vi "LB_SetCaptureGain.vi"(9 "Gain":u8=1 min=1 max=4, 10 "SamplingTime":T1, 11 "LB_COM_IN":refnum<visa-resource-name>="COM4") -> (2 "OK":bool)   [LabVIEW 2015, in "LBAnalyser.lvlib"]
uses:
  LBAnalyser.lvlib
  SamplingTime.ctl
  UartCOM/UARTCOM.lvlib
panel:
  out "error out":errorcluster caption="错误输出"
  in  "error in (no error)":errorcluster caption="错误输入（无错误）"
  # "1~4"
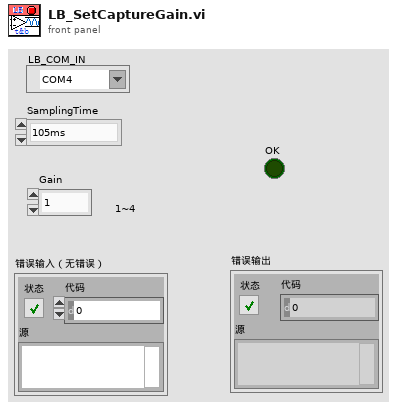
[diagram p1: front panel]
types:
  T1 = typedef "LBAnalyser.lvlib/SamplingTime.ctl" = enum8{"105ms", "120ms", "165ms", "270ms", "380ms", "880ms"}
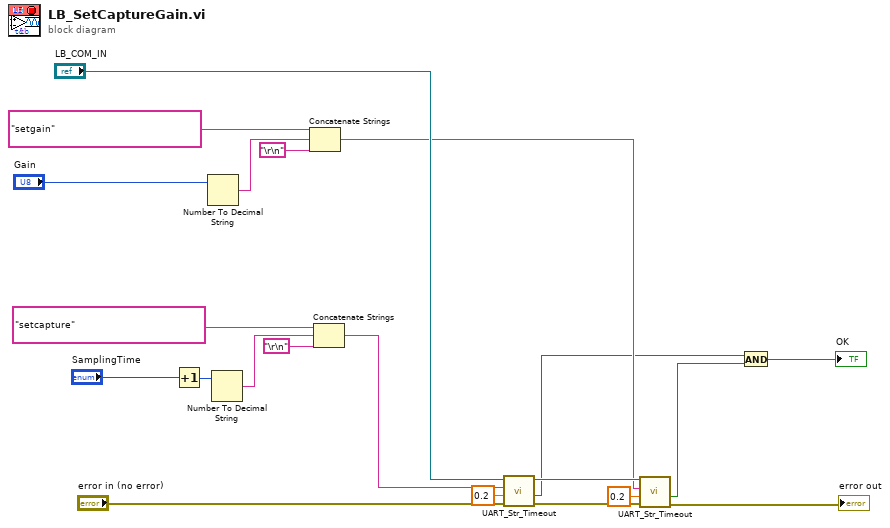
[diagram p0: block diagram]
diagram:
  n1 = Increment(x="SamplingTime") -> (x+1=w18:T1)
  n2 = Number To Decimal String(number="Gain") -> (decimal integer string=w12:string)  [unwired: 1 in]
  n3 = Number To Decimal String(number=w18) -> (decimal integer string=w16:string)  [unwired: 1 in]
  n4 = Concatenate Strings("setgain" ("写入字符串"), w12, "\r\n") -> (w5:string)
  n5 = Concatenate Strings("setcapture" ("写入字符串"), w16, "\r\n") -> (w14:string)
  n6 = call "UART_Str_Timeout.vi"("error in (no error)"="error in (no error)", "超时s"=0.2, "写入字符串"=w14, "BASE_COM"="LB_COM_IN") -> ("error out"=w7:errorcluster, "OK"=w3:bool, "BASE_COM_OUT"=w6:refnum<visa-resource-name>)  [unwired: 3 in, 2 out]
  n7 = call "UART_Str_Timeout.vi"("error in (no error)"=w7, "超时s"=0.2, "写入字符串"=w5, "BASE_COM"=w6) -> ("error out"=→"error out":errorcluster, "OK"=w2:bool)  [unwired: 3 in, 3 out]
  n8 = And(x=w3, y=w2) -> (x .and. y?=→"OK":bool)
